vi "putty.vi"() -> ()   [LabVIEW 2018]
panel:
  in  "Cammand need to be executed":string="pwd\nls\n"
  out "standard error":string
  out "standard output":string
  in  "operation (0:open)":T1(ring)=enum."replace or create"
  in  "-m":string=" -m "
  in  "Password":string=" labview==="
  in  "-pw":string=" -pw"
  in  "Operation":string=" -ssh"
  in  "Host name /ip":string="10.0.86.122"
  in  "Username":string="lvadmin"
  in  "Putty location":string="C:\\Users\\nitest\\Desktop\\putty[32bit].exe "
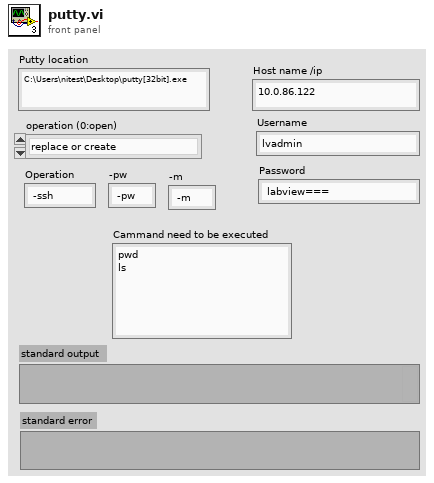
[diagram p1: front panel]
types:
  T1 = enum16{"open", "replace", "create", "open or create", "replace or create", "replace or create with confirmation"}
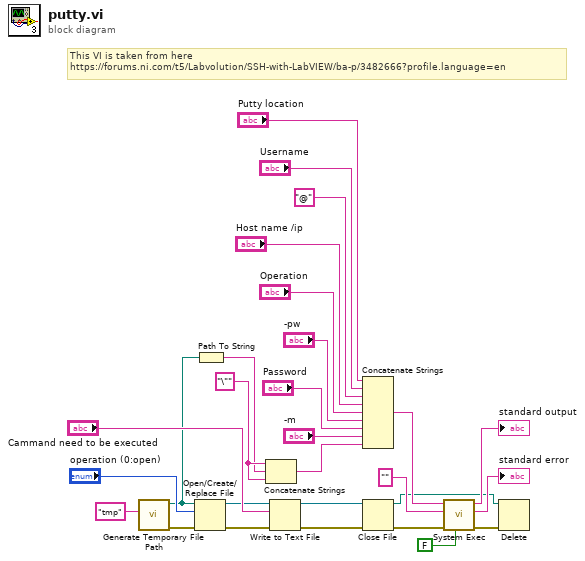
[diagram p0: block diagram]
diagram:
  w12 = "\"" ("string")
  # "This VI is taken from here \nhttps://forums.ni.com/t5/Labvolution/SSH-with-LabVIEW/ba-p/3482666?profile.language=en"
  n1 = call <vilib>:"Generate Temporary File Path.vi"("Temporary File Extension (tmp)"="tmp") -> ("error out"=w4:errorcluster, "Unique Temporary File Path"=w3:path)  [unwired: 9 in]
  n2 = Open/Create/Replace File(file path (use dialog)=w3, error in=w4, operation (0:open)="operation (0:open)") -> (refnum out=w10:refnum<file>, error out=w28:errorcluster)  [unwired: 3 in, 1 out]
  n3 = Path To String(path=w3) -> (string=w11:string)
  n4 = Concatenate Strings(w12, w11, w12) -> (w2:string)
  n5 = Write to Text File(file (use dialog)=w10, text="Cammand need to be executed", error in=w28) -> (refnum out=w15:refnum<file>, error out=w16:errorcluster)  [unwired: 1 in, 1 out]
  n6 = Concatenate Strings("Putty location", "Username", "@" ("string 3"), "Host name /ip", "Operation", "-pw", "Password", "-m", w2) -> (w17:string)
  n7 = Close File(refnum=w15, error in=w16) -> (path=w5:path, error out=w27:errorcluster)
  n8 = call <vilib>:"System Exec.vi"("run minimized? (F)"=FALSE, "error in (no error)"=w27, "standard input"="", "command line"=w17) -> ("error out"=w6:errorcluster, "standard error"=→"standard error":string, "standard output"=→"standard output":string)  [unwired: 4 in, 1 out]
  n9 = Delete(path (use dialog)=w5, error in=w6) -> ()  [unwired: 3 in, 3 out]
